vi "truncate.vi"(0 "input array 0":u16[](array[numeric]), 1 "size of array":u32, 5 "input array 1":u16[](array[numeric]), 7 "input array 2":u16[](array[numeric]), 9 "input array 3":u16[](array[numeric]), 11 "error in (no error)":errorcluster) -> (4 "output channel 0-3":u32[][](array[numeric]), 15 "error out":errorcluster)   [LabVIEW 2016]
doc: "array is truncated to only valid numbers"
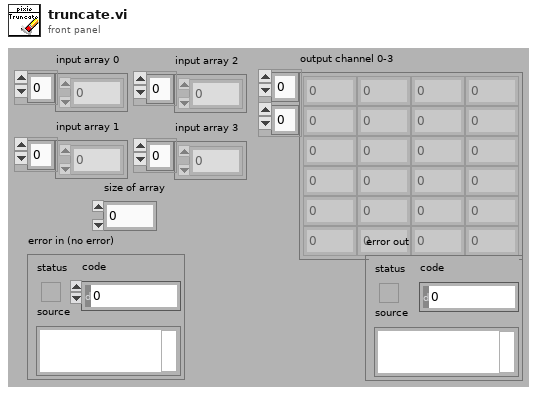
[diagram p1: front panel]
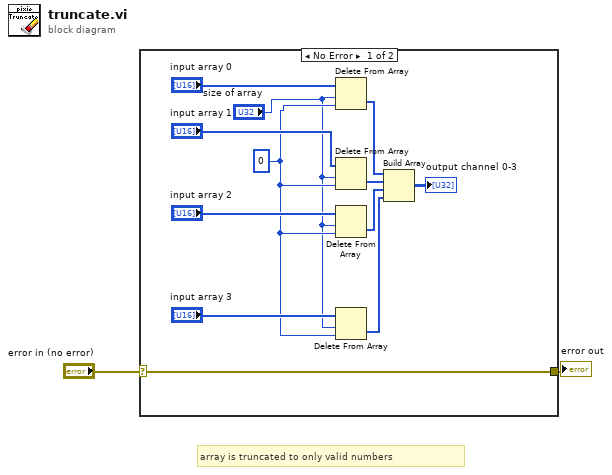
[diagram p0: block diagram]
diagram:
  # "array is truncated to only valid numbers"
  n1 = case shown="No Error" "error in (no error)" {
    selector: "error in (no error)" -> [w5 w15]
    tunnel: [w5 w15] -> w1
    frame No Error {
      w4 = i16 0 ("Numeric")
      n2 = Delete From Array(array="input array 0", length="size of array", index=w4) -> (deleted portion=w11:u16[])  [unwired: 1 out]
      n3 = Delete From Array(array="input array 1", length="size of array", index=w4) -> (deleted portion=w12:u16[])  [unwired: 1 out]
      n4 = Delete From Array(array="input array 2", length="size of array", index=w4) -> (deleted portion=w13:u16[])  [unwired: 1 out]
      n5 = Delete From Array(array="input array 3", length="size of array", index=w4) -> (deleted portion=w14:u16[])  [unwired: 1 out]
      n6 = Build Array(w11, w12, w13, w14) -> (→"output channel 0-3":u16[][])
    }
    frame Error {
    }
  }
  "error out" <- w1
